vi "GMLAN ReadMemoryByAddress.vi"(7 "MemoryAddressLength":enum8{"Two", "Three", "Four"}(ring), 8 "error in (no error)":errorcluster, 9 "MemorySize":u16, 10 "MemoryAddress":u32, 11 "diag ref in":T1) -> (0 "error out":errorcluster, 1 "success?":bool, 2 "data out":u8[](array[numeric]), 3 "diag ref out":T1)   [LabVIEW 2013, in "GMLAN.lvlib"]
uses:
  GMLAN.lvlib
  <vilib>/Automotive Diagnostic Command Set/Diagnostic Transport.llb/Diag Reference.ctl
  <vilib>/Automotive Diagnostic Command Set/Diagnostic Transport.llb/Transport Protocol Selector.ctl
  <vilib>/Automotive Diagnostic Command Set/Diagnostic Transport.llb/Diag CAN Frame Log.ctl
  <vilib>/addons/Automotive Diagnostic Command Set/NI_Automotive Diagnostic Command Set.lvlib
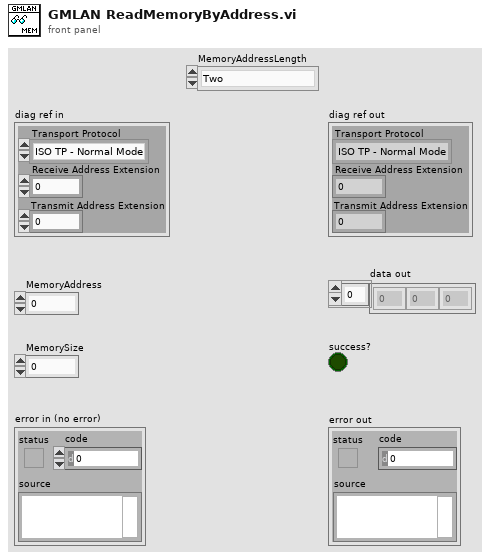
[diagram p1: front panel]
types:
  T1 = typedef "NI_Automotive Diagnostic Command Set.lvlib/Diag Reference.ctl" = cluster{"Diag CAN Handle":u32, "Transport Protocol":T2, "Receive Address Extension":u8, "Transmit Address Extension":u8, "Receive CAN Id":u32, "Transmit CAN Id":u32, "Diag CAN Queue":refnum<queue>, "Log Frames ?":bool, "My TP Address":u8, "Other TP Address":u8, "T1":u16, "T2":u16, "T3":u16, "T4":u16, "Tx SN":u8, "Block Size":u8, "Rx SN":u8, "VW TP Initialized?":bool, "Tx block no":u8, "baud rate":u32, "Interface":string, "Channel Diag CAN Handle":u32, "UDP Connection ID":refnum<k16>, "TCP Connection ID":refnum<k5>, "Target IP Addr":u32, "Source Address":u16, "Target Address":u16, "Send Header NACK?":bool, "DLL Handle":u32, "NAD":u8}
  T2 = typedef "NI_Automotive Diagnostic Command Set.lvlib/Transport Protocol Selector.ctl" = enum16{"ISO TP - Normal Mode", "ISO TP - Mixed Mode", "VW TP 2.0", "Diagnostics on IP", "ISO TP LIN"}
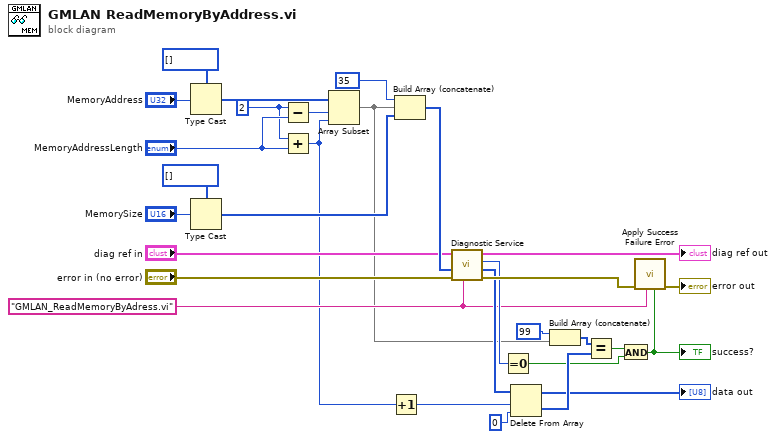
[diagram p0: block diagram]
diagram:
  w4 = 2 ("index")
  w13 = "GMLAN_ReadMemoryByAdress.vi" ("error source")
  n1 = Type Cast(type=u8[] [], x="MemoryAddress") -> (*(type *) &x=w7:u8[])
  n2 = Type Cast(type=u8[] [], x="MemorySize") -> (*(type *) &x=w12:u8[])
  n3 = Subtract(x=w4, y="MemoryAddressLength") -> (x-y=w5:i32)
  n4 = Add(x=w4, y="MemoryAddressLength") -> (x+y=w2:i32)
  n5 = Array Subset(array=w7, index=w5, length=w2) -> (w3:u8[])
  n6 = Increment(x=w2) -> (x+1=w1:i32)
  n7 = Build Array (concatenate)(u8 35 ("element"), w3, w12) -> (w26:u8[])
  n8 = call <vilib>:"Diagnostic Service.vi"("error source"=w13, "error in (no error)"="error in (no error)", "data in"=w26, "diag ref in"="diag ref in") -> ("error out"=w28:errorcluster, "data out"=w21:u8[], "error code"=w25:u8, "diag ref out"=→"diag ref out":T1)  [unwired: 2 in, 2 out]
  n9 = Equal To 0?(x=w25) -> (x = 0?=w19:bool)
  n10 = Delete From Array(array=w21, length=w1, index=0) -> (deleted portion=w20:u8[], array with subset deleted=→"data out":u8[])
  n11 = Build Array (concatenate)(u8 99 ("element"), w3) -> (w22:u8[])
  n12 = Equal?(x=w22, y=w20) -> (x = y?=w17:bool)
  n13 = And(x=w17, y=w19) -> (x .and. y?=w14:bool)
  "success?" <- w14
  n14 = call <vilib>:"Apply Success Failure Error.vi"("success code"=w14, "error source"=w13, "error in (no error)"=w28) -> ("error out"=→"error out":errorcluster)  [unwired: 8 out]
